vi "Reorder Poles and Residues.vi"(9 "Poles In":cdb[](array[numeric]), 10 "Residues In":cdb[][](array[numeric]), 11 "Multiplicity In":i32[](array[numeric])) -> (0 "error":i32, 1 "Poles Out":cdb[](array[numeric]), 2 "Residues Out":cdb[][](array[numeric]), 3 "Multiplicity Out":i32[](array[numeric]))   [LabVIEW 2017, in "NI_AALPro.lvlib"]
uses:
  NI_AALPro.lvlib
  Leja Order Roots (CDB).vi
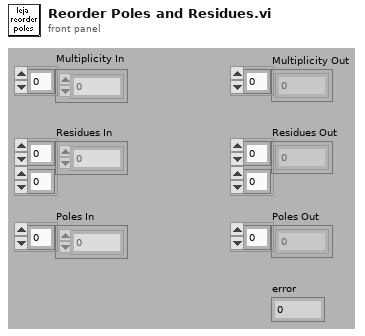
[diagram p1: front panel]
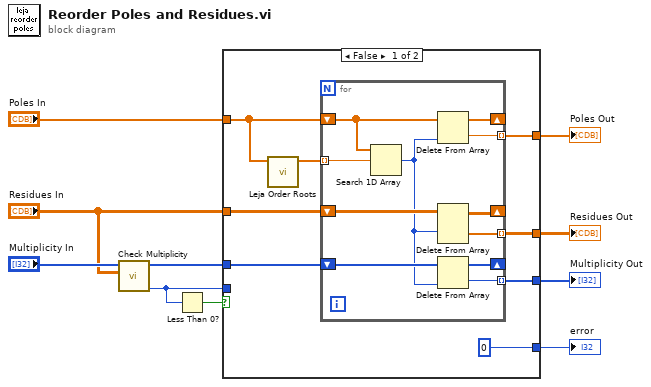
[diagram p0: block diagram]
diagram:
  n1 = call "Check Multiplicity.vi"("Residues"="Residues In", "Multiplicity In"="Multiplicity In") -> ("error"=w8:i32, "Multiplicity Out"=w7:i32[])  [unwired: 8 in]
  n2 = Less Than 0?(x=w8) -> (x < 0?=w9:bool)
  n3 = case shown="False" w9 {
    tunnel: w8 -> [_ w30]
    tunnel: w7 -> [w17 _]
    tunnel: "Residues In" -> [w18 _]
    tunnel: "Poles In" -> [w16 _]
    tunnel: [w14 _] -> w4
    tunnel: [w13 _] -> w3
    tunnel: [w12 _] -> w2
    tunnel: [0 ("error") w30] -> w1
    frame False {
      n4 = call-poly "Leja Order Roots.vi"("Roots"=w16) -> ("Roots of Leja Order"=w15:cdb[])  [unwired: 10 in]
      n5 = for {
        tunnel: w15 -> [w29] mode=indexing
        shift-right: [w27] -> _
        shift-left: w16 -> [w28]
        shift-right: [w24] -> _
        shift-left: w18 -> [w25]
        shift-right: [w21] -> _
        shift-left: w17 -> [w22]
        tunnel: [w26] -> w14 mode=indexing
        tunnel: [w23] -> w13 mode=indexing
        tunnel: [w20] -> w12 mode=indexing
        n6 = Search 1D Array(1D array=w28, element=w29) -> (index of element=w19:i32)  [unwired: 1 in]
        n7 = Delete From Array(array=w28, index=w19) -> (deleted portion=w26:cdb, array with subset deleted=w27:cdb[])  [unwired: 1 in]
        n8 = Delete From Array(array=w25, index (row)=w19) -> (deleted portion=w23:cdb[], array with subset deleted=w24:cdb[][])  [unwired: 2 in]
        n9 = Delete From Array(array=w22, index=w19) -> (deleted portion=w20:i32, array with subset deleted=w21:i32[])  [unwired: 1 in]
      }
    }
    frame True {
    }
  }
  "error" <- w1
  "Multiplicity Out" <- w2
  "Residues Out" <- w3
  "Poles Out" <- w4
